vi "FTW-Actor-ConfigureTiming-Proactor-WallClock.vi"(0 "FTW Actor Instance":refnum<class "FTW-Actor-Instance.lvclass">, 1 "Preempt Job Queue on Timeout":bool, 5 "Timeout Period":dbl=1.0 format="%#.6psec", 7 "Timeout Offset from Clock Multiple":dbl format="%#.6psec", 9 "Iterations (-1 to loop forever)":i32=-1 format="%d iterations", 11 "error in":errorcluster) -> (4 "FTW Actor Instance out":refnum<class "FTW-Actor-Instance.lvclass">, 15 "error out":errorcluster)   [LabVIEW 2015, in "FTW-Actor-Instance.lvclass"]
uses:
  FTW-Actor-Instance.lvclass
panel:
  # "Inputs"
  # "Outputs"
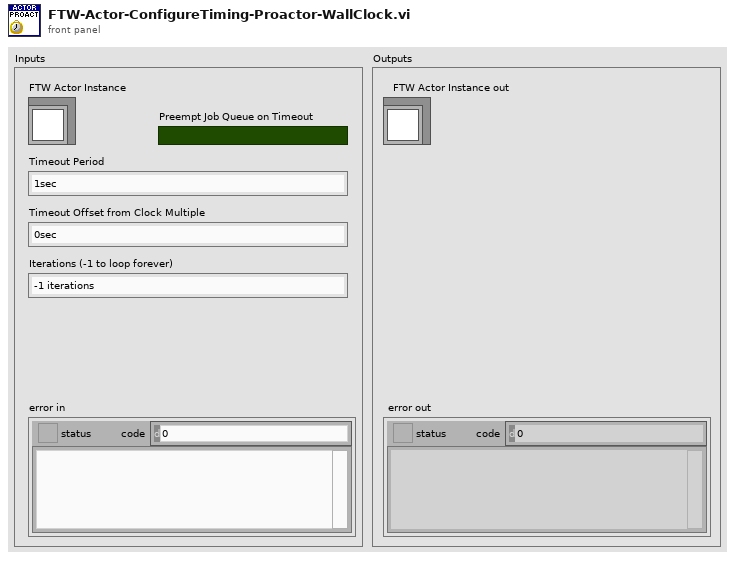
[diagram p1: front panel]
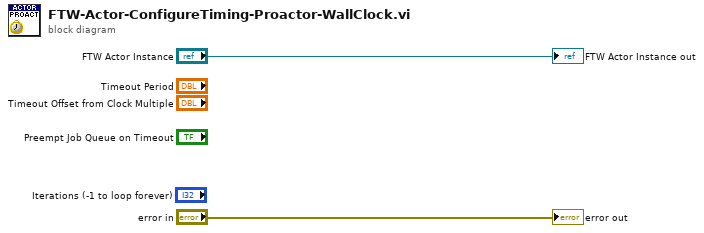
[diagram p0: block diagram]
diagram:
  "error out" <- "error in"
  "FTW Actor Instance out" <- "FTW Actor Instance"
